vi "SetParam.vi"(8 "error in (no error)":errorcluster, 11 "Microscope in":refnum<class "Microscope.lvclass">) -> (0 "error out":errorcluster, 3 "Microscope out":refnum<class "Microscope.lvclass">)   [LabVIEW 2012, in "Microscope.lvclass"]
uses:
  classes/Microscope.lvclass
  typedefs/MicroscopeEvent.ctl
  classes/Microscope.lvclass/Microscope.ctl
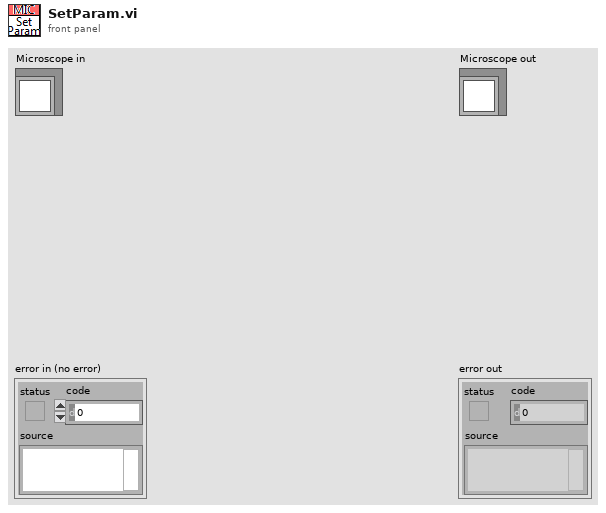
[diagram p1: front panel]
types:
  T1 = typedef "MicroscopeEvent.ctl" = enum16{"M.Wait", "M.RunRotation", "M.Flush", "M.Init", "M.InitStage", "M.InitImageData", "M.ReinitImageData", "M.ReinitImageParams", "M.GetSetParams", "M.InitFastHardware", "M.Pre-Acquire", "M.Acquire", "M.PostAcquire", "M.StopAcquire", "M.SetAcqStatusTrue", "M.SetAcqStatusFalse", "M.ClearImageData", "M.MoveStageDiscrete", "M.MoveStageToTarget1", "M.MoveStageToTarget2", "M.MoveStageToTarget3", "M.OpenShutters", "M.CloseShutters", "M.StartAcquireSequence", "M.ChangeParameters", "M.OpenStokes", "M.OpenPump", "M.RunSW"}
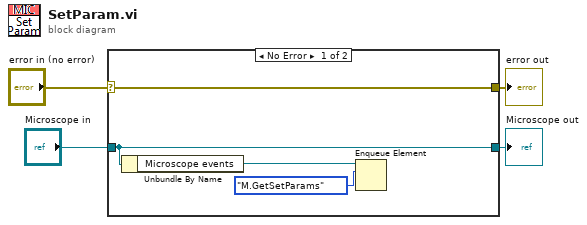
[diagram p0: block diagram]
diagram:
  n1 = case shown="No Error" "error in (no error)" {
    selector: "error in (no error)" -> [w8 w10]
    tunnel: [w8 w10] -> w3
    tunnel: [w7 w9] -> w1
    tunnel: "Microscope in" -> [w7 w9]
    frame No Error {
      n2 = Unbundle By Name(w7) -> ("Microscope events"=w5:refnum<queue>)
      n3 = Enqueue Element(queue=w5, element=MicroscopeEvent."M.GetSetParams") -> ()  [unwired: 2 in, 3 out]
    }
    frame Error {
    }
  }
  "error out" <- w3
  "Microscope out" <- w1
